vi "generateTempFile.vi"(8 "error in (no error)":errorcluster, 11 "MS-Excel in":refnum<class "MS-Excel.lvclass">) -> (0 "error out":errorcluster, 2 "Temporary File Path":path, 3 "MS-Excel out":refnum<class "MS-Excel.lvclass">)   [LabVIEW 2017, in "LabVIEW NPOI.lvlib" / "MS-Excel.lvclass"]
uses:
  MS-Excel.lvclass
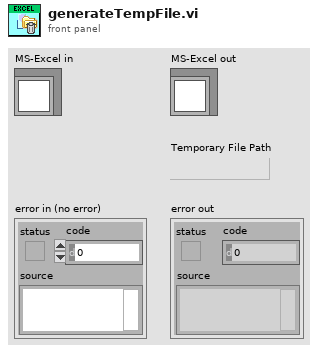
[diagram p1: front panel]
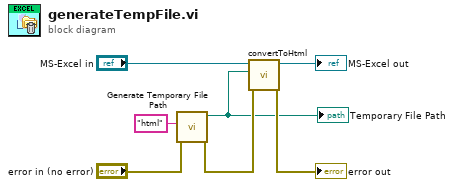
[diagram p0: block diagram]
diagram:
  n1 = call <vilib>:"Generate Temporary File Path.vi"("error in (no error)"="error in (no error)", "Temporary File Extension (tmp)"="html") -> ("error out"=w4:errorcluster, "Unique Temporary File Path"=w1:path)  [unwired: 8 in]
  "Temporary File Path" <- w1
  n2 = call-dynamic "convertToHtml.vi"("error in (no error)"=w4, "HTML File Path"=w1, "MS-Excel in"="MS-Excel in") -> ("error out"=→"error out":errorcluster, "MS-Excel out"=→"MS-Excel out":refnum<class "MS-Excel.lvclass">)  [unwired: 7 in]
